vi "CRYFlatten Start.vi"(11 "Start":T1) -> (3 "Start flattened":string)   [LabVIEW 2013]
uses:
  Typedef Control/CRYStart Cluster.ctl
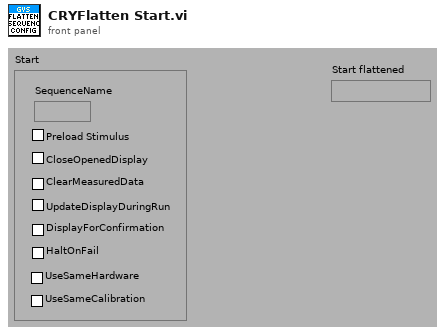
[diagram p1: front panel]
types:
  T1 = typedef "CRYStart Cluster.ctl" = cluster{"SequenceName":string, "Preload Stimulus":bool, "CloseOpenedDisplay":bool, "ClearMeasuredData":bool, "UpdateDisplayDuringRun":bool, "DisplayForConfirmation":bool, "HaltOnFail":bool, "UseSameHardware":bool, "UseSameCalibration":bool}
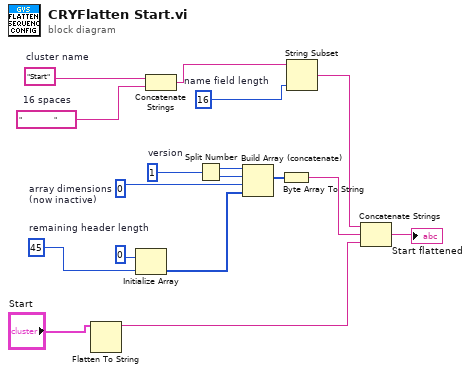
[diagram p0: block diagram]
diagram:
  w3 = u8 0  # array dimensions (now inactive)
  w6 = 16  # name field length
  w7 = "                "  # 16 spaces
  w8 = "Start"  # cluster name
  w13 = 45  # remaining header length
  w17 = u16 1  # version
  n1 = Flatten To String(anything="Start") -> (data string=w2:string)  [unwired: 1 in, 4 out]
  n2 = Initialize Array(u8 0, w13) -> (w9:u8[])
  n3 = Concatenate Strings(w8, w7) -> (w5:string)
  n4 = Split Number(x=w17) -> (hi(x)=w16:u8, lo(x)=w15:u8)
  n5 = Build Array (concatenate)(w16, w15, w3, w9) -> (w12:u8[])
  n6 = Byte Array To String(unsigned byte array=w12) -> (string=w10:string)
  n7 = String Subset(string=w5, length (rest)=w6) -> (substring=w4:string)  [unwired: 1 out]
  n8 = Concatenate Strings(w4, w10, w2) -> (→"Start flattened":string)
